vi "CVT Double StaticWrite.vi"(3 "error in (no error)":errorcluster, 4 "Value":dbl, 5 "Tag Name":string) -> (0 "error out":errorcluster)   [LabVIEW 2016]
uses:
  <vilib>/NI/Current Value Table/DataTypes/Double_Static Write.vi
  <vilib>/NI/Current Value Table/Type to Enum.vi
  <vilib>/NI/Current Value Table/DataTypes/Double_Type To Enum.vi
  <vilib>/NI/Current Value Table/Memory Block.vi
  <vilib>/NI/Current Value Table/DataTypes/Double_Memory Block.vi
  <vilib>/NI/Current Value Table/FGVs/Tag Memory.vi
  <vilib>/NI/Current Value Table/Current Value Table.lvlib
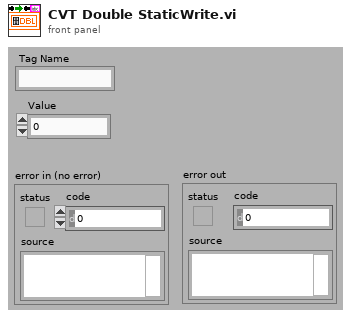
[diagram p1: front panel]
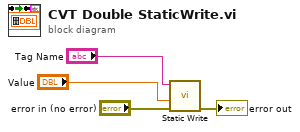
[diagram p0: block diagram]
diagram:
  n1 = call-poly <vilib>:"Static Write.vi"("error in (no error)"="error in (no error)", "Value"="Value", "Tag Name"="Tag Name") -> ("error out"=→"error out":errorcluster)  [unwired: 8 in]
